vi "RSZVB File Catalog.vi"(8 "error in (no error)":errorcluster {"code" format="%.0x"}, 10 "Directory (D:\\user\\data)":string="D:\\user\\data", 11 "VISA session":refnum<visa-resource-name>) -> (0 "error out":errorcluster {"code" format="%.0x"}, 2 "Catalog":string, 3 "dup VISA session":refnum<visa-resource-name>)   [LabVIEW 2011]
doc: "This VI reads the indicated directory. According to DOS convention, wild card characters can be entered in order to query e.g. a list of all files of a certain type.\n\nRemote-control command(s):\nMMEMory:CDIRectory '<directory_name>'\nMMEMory:CATalog?\nMMEMory:CATalog:ALL?"
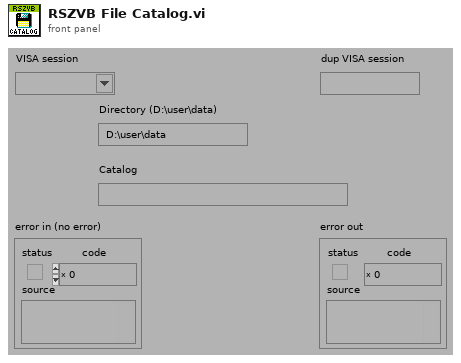
[diagram p1: front panel]
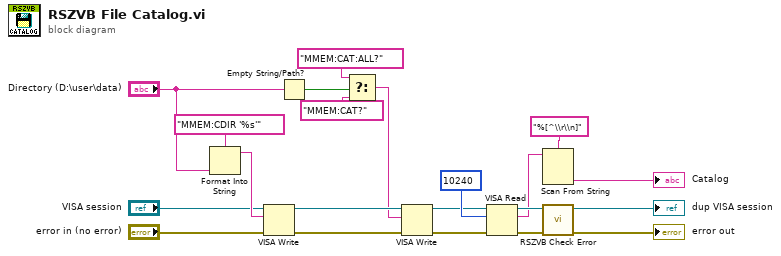
[diagram p0: block diagram]
diagram:
  n1 = Format Into String(format string="MMEM:CDIR '%s'", "Directory (D:\\user\\data)") -> (resulting string=w20:string)  [unwired: 2 in, 1 out]
  n2 = VISA Write(VISA resource name="VISA session", write buffer=w20, error in (no error)="error in (no error)") -> (VISA resource name out=w15:refnum<visa-resource-name>, error out=w16:errorcluster)  [unwired: 1 out]
  n3 = Empty String/Path?(string/path="Directory (D:\\user\\data)") -> (empty?=w7:bool)
  n4 = Select(t="MMEM:CAT:ALL?", s=w7, f="MMEM:CAT?") -> (s? t:f=w4:string)
  n5 = VISA Write(VISA resource name=w15, write buffer=w4, error in (no error)=w16) -> (VISA resource name out=w18:refnum<visa-resource-name>, error out=w17:errorcluster)  [unwired: 1 out]
  n6 = VISA Read(VISA resource name=w18, byte count=u32 10240 ("byte count (0)"), error in (no error)=w17) -> (VISA resource name out=w12:refnum<visa-resource-name>, read buffer=w1:string, error out=w9:errorcluster)  [unwired: 1 out]
  n7 = Scan From String(format string="%[^\\r\\n]", input string=w1) -> (output 1=→"Catalog":string)  [unwired: 3 in, 3 out]
  n8 = call "RSZVB Check Error.vi"("error in (no error)"=w9, "VISA session"=w12) -> ("error out"=→"error out":errorcluster, "dup VISA session"=→"dup VISA session":refnum<visa-resource-name>)  [unwired: 8 in]
